vi "Filename checker2 (SubVI).vi"(6 "Append? In":bool, 9 "Path in":path) -> (0 "Append? Out":bool, 3 "Path out":path)   [LabVIEW 2017, in "Fridge Software v2.1.lvlib"]
uses:
  Fridge Software v2.1.lvlib
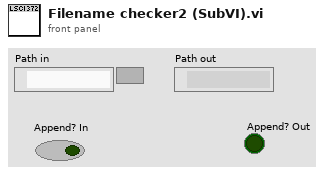
[diagram p1: front panel]
types:
  T1 = enum16{"Left Button", "Center Button", "Right Button", "Window Close"}
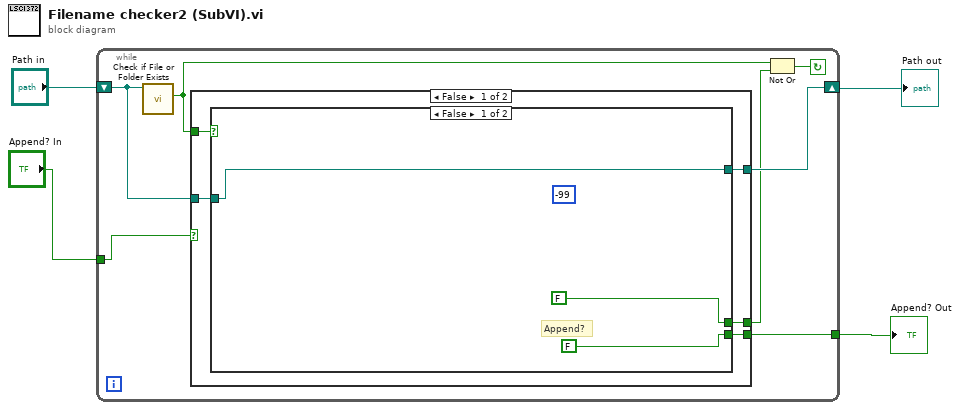
[diagram p0: block diagram]
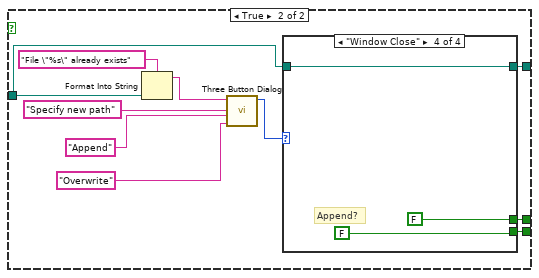
[diagram p2: hidden frame]
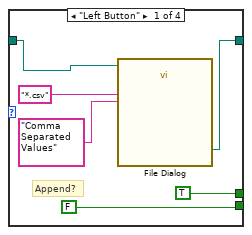
[diagram p3: hidden frame]
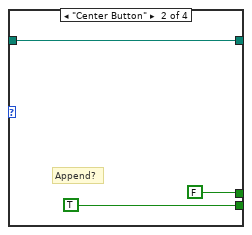
[diagram p4: hidden frame]
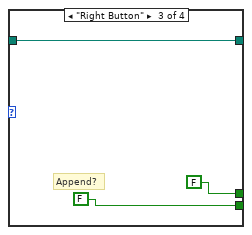
[diagram p5: hidden frame]
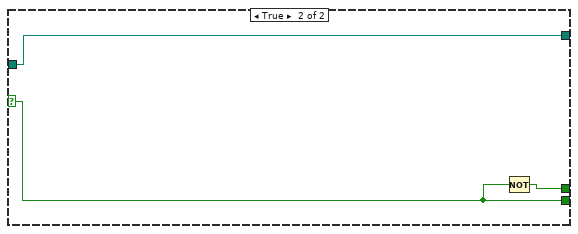
[diagram p6: hidden frame]
diagram:
  n1 = while {
    shift-right: [w9] -> w3
    shift-left: "Path in" -> [w11]
    tunnel: [w6] -> w4
    tunnel: "Append? In" -> [w5]
    stop <- w10 continue-if-true
    n2 = call <vilib>:"Check if File or Folder Exists.vi"("path"=w11) -> ("file or folder exists?"=w7:bool)  [unwired: 8 in, 2 out]
    n3 = case shown="False" w5 {
      selector: w5 -> [_ w46]
      tunnel: w11 -> [w16 w47]
      tunnel: [w15 w47] -> w9
      tunnel: [w14 w45] -> w8
      tunnel: w7 -> [w13 _]
      tunnel: [w12 w46] -> w6
      frame False {
        n4 = case shown="False" w13 {
          tunnel: w16 -> [w19 w23]
          tunnel: [w19 w22] -> w15
          tunnel: [FALSE w21] -> w14
          tunnel: [FALSE w20] -> w12
          frame False {
            (unwired) -99
            # "Append?"
          }
          frame True {
            n5 = Format Into String(format string="File \"%s\" already exists", w23) -> (resulting string=w25:string)  [unwired: 2 in, 1 out]
            n6 = call <vilib>:"Three Button Dialog.vi"("Right Button Text (\"Cancel\")"="Overwrite", "Center Button Text (\"No\")"="Append", "Left Button Text (\"Yes\")"="Specify new path", "message"=w25) -> ("Which Button?"=w24:T1)  [unwired: 7 in]
            n7 = case shown="\"Window Close\"" w24 {
              tunnel: w23 -> [w35 w38 w41 w44]
              tunnel: [w32 w38 w41 w44] -> w22
              tunnel: [TRUE FALSE FALSE FALSE] -> w21
              tunnel: [FALSE TRUE FALSE FALSE] -> w20
              frame "Left Button" {
                # "Append?"
                n8 = call "File Dialog"("start path"=w35, "pattern (all files)"="*.csv", "pattern label"="Comma Separated Values") -> ("selected path"=w32:path)  [unwired: 9 in, 3 out]
              }
              frame "Center Button" {
                # "Append?"
              }
              frame "Right Button" {
                # "Append?"
              }
              frame "Window Close" {
                # "Append?"
              }
            }
          }
        }
      }
      frame True {
        n9 = Not(x=w46) -> (.not. x?=w45:bool)
      }
    }
    n10 = Not Or(1:w8, 2:w7) -> (0:w10:bool)
  }
  "Append? Out" <- w4
  "Path out" <- w3
